vi "Write DAC Voltage - Single DUT.vi"(0 "Channel (0-5)":u32, 5 "Voltage":dbl format="%.3f V", 7 "Vref (-1: Unchanged)":dbl=-1.0 format="%.3f V", 11 "error in":errorcluster, 12 "Log (T)":bool=TRUE, 13 "DUT":T2, 14 "FPGA":T1) -> (4 "Data Out":string, 15 "error out":errorcluster)   [LabVIEW 2017, in "Host SRL.lvlib"]
uses:
  Host SRL.lvlib
  Type Defs/WSVCAP SHL DUT Number Enum.ctl
  Type Defs/WSVCAP SHL FPGA Enum.ctl
  Type Defs/Cap and DAC Table Manager Operation Enum.ctl
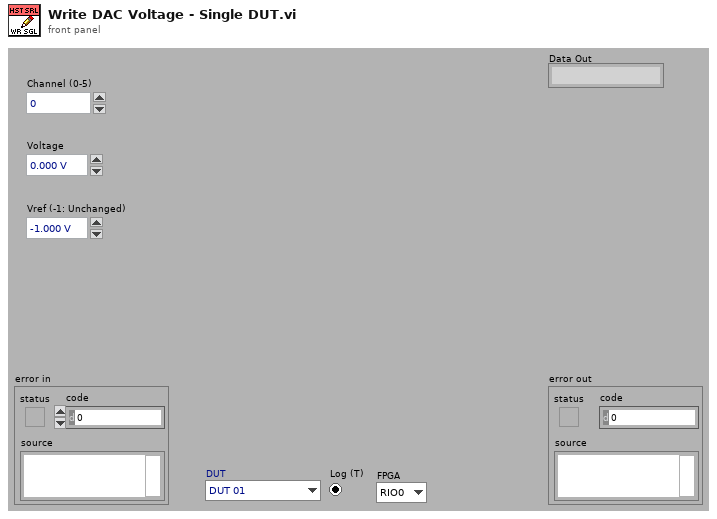
[diagram p1: front panel]
types:
  T1 = typedef "WSVCAP SHL FPGA Enum.ctl" = enum16{"RIO0", "RIO1"}
  T2 = typedef "WSVCAP SHL DUT Number Enum.ctl" = enum16{"DUT 01", "DUT 02", "DUT 03", "DUT 04", "DUT 05", "DUT 06", "DUT 07", "DUT 08", "DUT 09", "DUT 10", "DUT 11", "DUT 12", "DUT 13", "DUT 14", "DUT 15", "DUT 16", "DUT 17", "DUT 18", "DUT 19", "DUT 20", "DUT 21", "DUT 22", "DUT 23", "DUT 24"}
  T3 = typedef "Cap and DAC Table Manager Operation Enum.ctl" = enum16{"Initialize", "Add Single DAC", "Add All DAC", "Add All DUT Single DAC", "Add All Cap", "Get Status"}
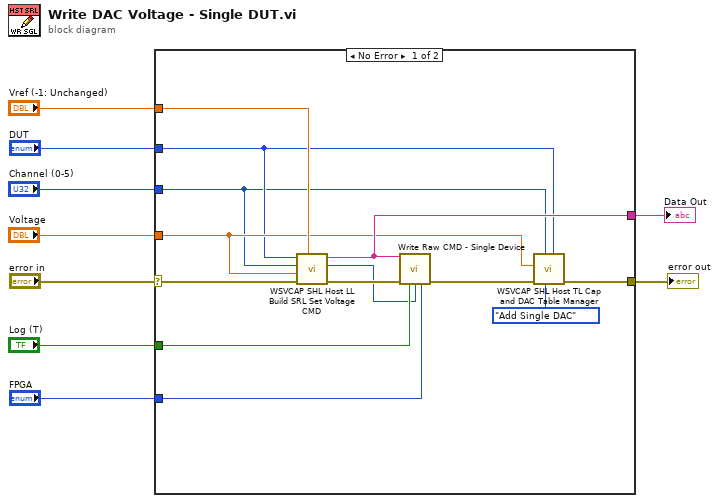
[diagram p0: block diagram]
diagram:
  n1 = case shown="No Error" "error in" {
    selector: "error in" -> [w19 _]
    tunnel: [w14 _] -> w9
    tunnel: "DUT" -> [w11 _]
    tunnel: "Log (T)" -> [w20 _]
    tunnel: "FPGA" -> [w21 _]
    tunnel: [w22 _] -> w4
    tunnel: "Channel (0-5)" -> [w10 _]
    tunnel: "Voltage" -> [w13 _]
    tunnel: "Vref (-1: Unchanged)" -> [w17 _]
    frame No Error {
      n2 = call "WSVCAP SHL Host LL Build SRL Set Voltage CMD.vi"("Vref (-1: Unchanged)"=w17, "error in (no error)"=w19, "Voltage (-1: Use Data Out)"=w13, "Channel (0-5)"=w10, "DUT"=w11) -> ("error out"=w18:errorcluster, "Dev Idx (0-5)"=w16:u32, "Raw CMD [Str]"=w22:string)  [unwired: 2 in, 2 out]
      n3 = call "Write Raw CMD - Single Device.vi"("Data Out"=w22, "error in"=w18, "Log (T)"=w20, "Device Idx (0-5)"=w16, "FPGA"=w21) -> ("error out"=w15:errorcluster)  [unwired: 10 in]
      n4 = call "WSVCAP SHL Host TL Cap and DAC Table Manager.vi"("DUT"=w11, "Operation"=Cap_and_DAC_Table_Manager_Operation_Enum."Add Single DAC", "Channel (0-5)"=w10, "Error In"=w15, "Voltage"=w13) -> ("Error Out"=w14:errorcluster)  [unwired: 5 in, 1 out]
    }
    frame Error {
    }
  }
  "error out" <- w9
  "Data Out" <- w4
